vi "Add Selected Ctrl Properties.vi"(11 "Data Cluster In":T1) -> (0 "New data?":bool, 3 "Data Cluster out":T1)   [LabVIEW 2021, in "Control Property Tree.lvlib"]
uses:
  Control Property Tree.lvlib
  Module Data--cluster.ctl
  Ctrl Properties Map Data.ctl
  Property array.ctl
  Selected Ctrls - List of Controls.ctl
  Selected Ctrls - List of Properties.ctl
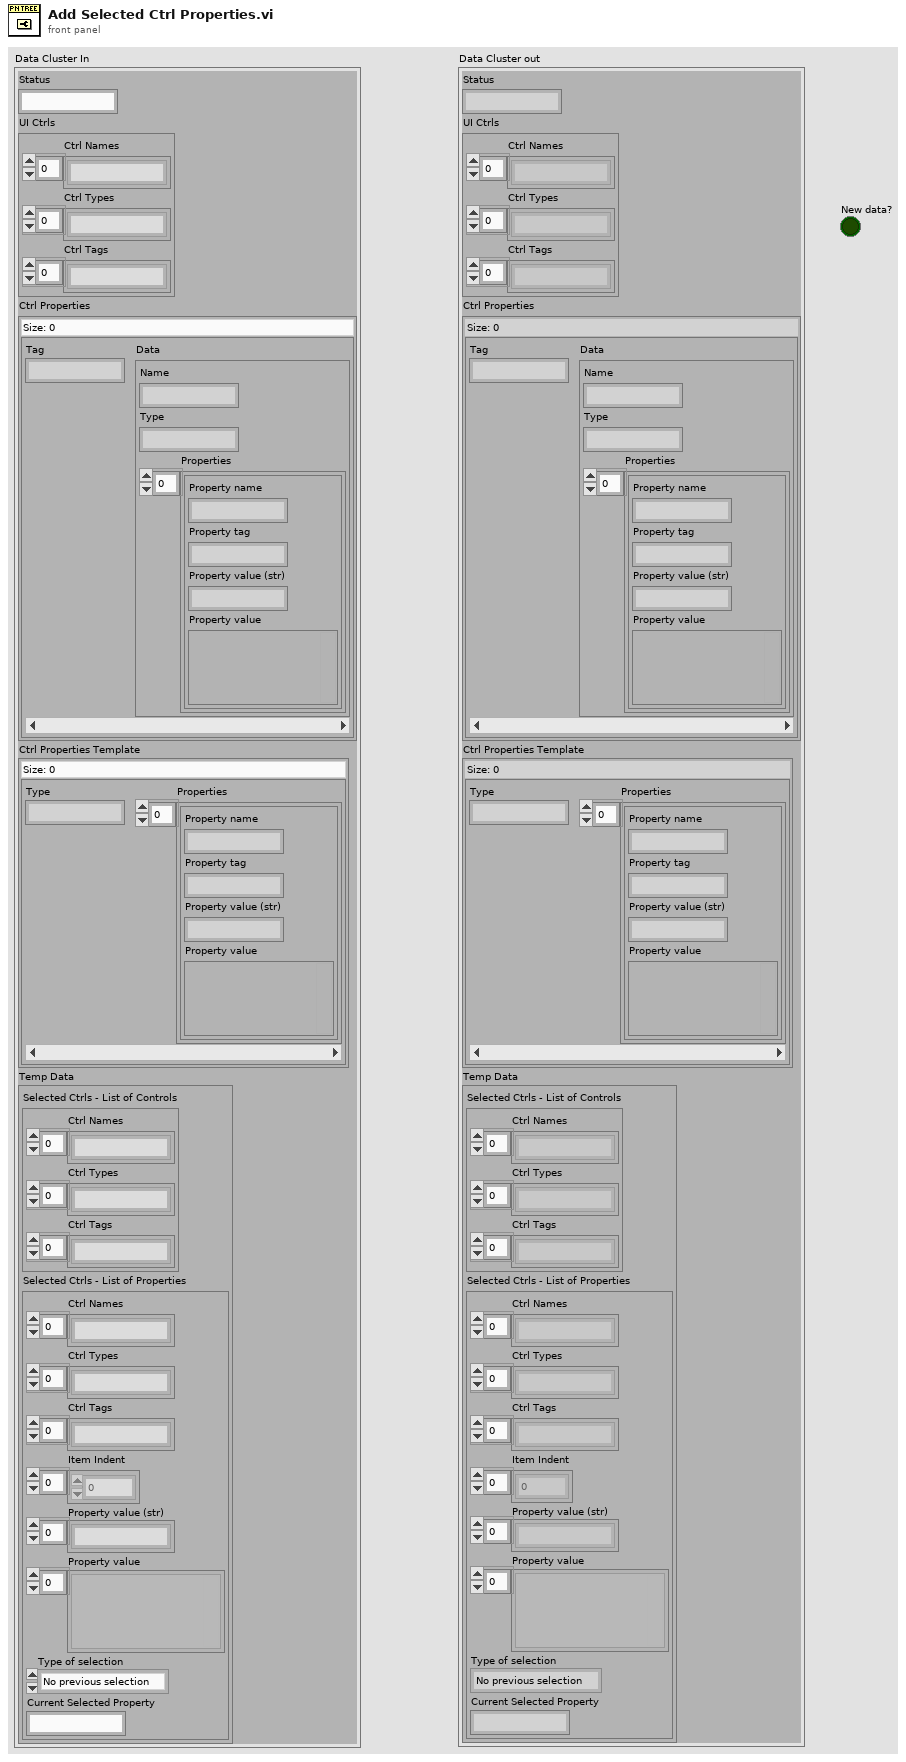
[diagram p1: front panel]
types:
  T1 = typedef "Control Property Tree.lvlib/Module Data--cluster.ctl" = cluster{"Status":string, "UI Ctrls":cluster{"Ctrl Names":string[], "Ctrl Types":string[], "Ctrl Tags":string[]}, "Ctrl Properties":map{string, T2}, "Ctrl Properties Template":map{string, T3}, "Temp Data":cluster{"Selected Ctrls - List of Controls":T4, "Selected Ctrls - List of Properties":T5}}
  T2 = typedef "Control Property Tree.lvlib/Ctrl Properties Map Data.ctl" = cluster{"Name":string, "Type":string, "Properties":T3}
  T3 = typedef "Control Property Tree.lvlib/Property array.ctl" = cluster{"Property name":string, "Property tag":string, "Property value (str)":string, "Property value":variant}[]
  T4 = typedef "Control Property Tree.lvlib/Selected Ctrls - List of Controls.ctl" = cluster{"Ctrl Names":string[], "Ctrl Types":string[], "Ctrl Tags":string[]}
  T5 = typedef "Control Property Tree.lvlib/Selected Ctrls - List of Properties.ctl" = cluster{"Ctrl Names":string[], "Ctrl Types":string[], "Ctrl Tags":string[], "Item Indent":i32[], "Property value (str)":string[], "Property value":variant[], "Type of selection":enum16{"No previous selection", "Control selected", "Property selected"}, "Current Selected Property":string}
  T6 = cluster{"Property name":string, "Property tag":string, "Property value (str)":string, "Property value":variant}
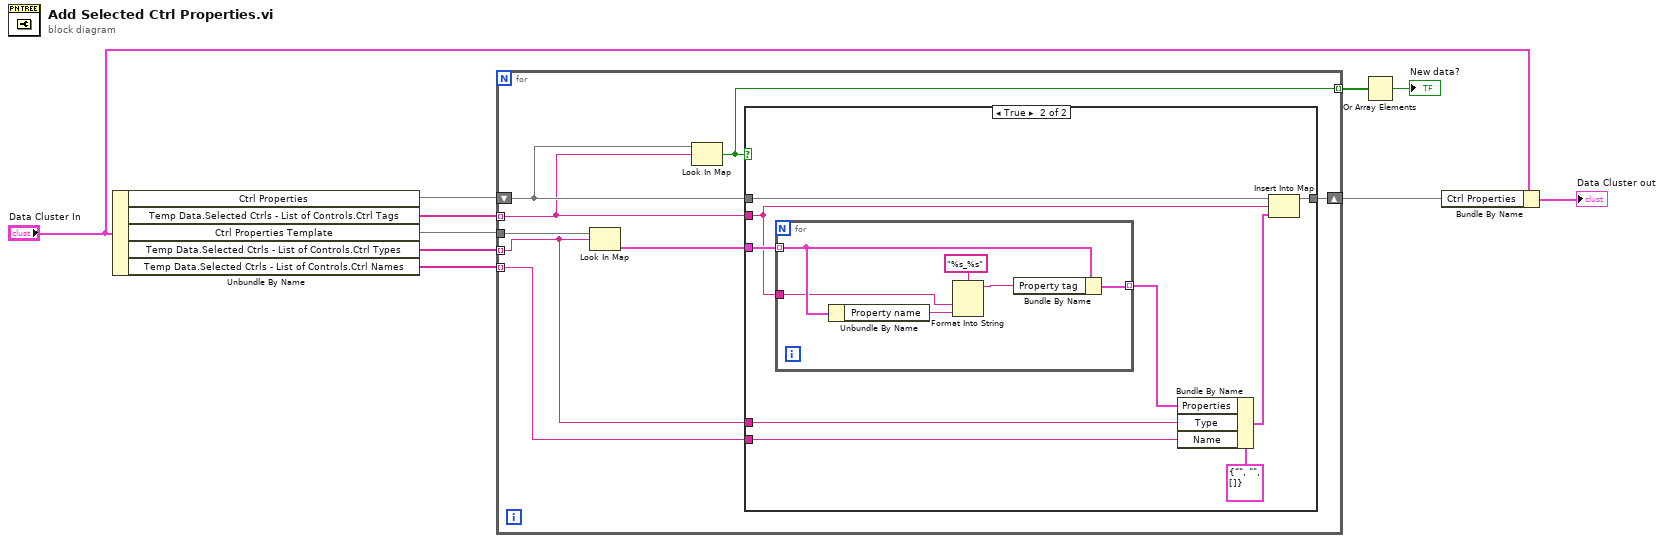
[diagram p0: block diagram]
diagram:
  n1 = Unbundle By Name("Data Cluster In") -> ("Ctrl Properties"=w7:map{string, T2}, "Temp Data.Selected Ctrls - List of Controls.Ctrl Tags"=w6:string[], "Ctrl Properties Template"=w8:map{string, T3}, "Temp Data.Selected Ctrls - List of Controls.Ctrl Types"=w10:string[], "Temp Data.Selected Ctrls - List of Controls.Ctrl Names"=w9:string[])
  n2 = for {
    tunnel: w10 -> [w16] mode=indexing
    tunnel: w9 -> [w15] mode=indexing
    tunnel: w8 -> [w18]
    tunnel: w6 -> [w12] mode=indexing
    shift-right: [w14] -> w4
    shift-left: w7 -> [w13]
    tunnel: [w11] -> w2 mode=indexing
    n3 = Look In Map(map=w18, key=w16) -> (value=w17:T3)  [unwired: 1 in, 1 out]
    n4 = Look In Map(map=w13, key=w12) -> (key not found?=w11:bool)  [unwired: 1 in, 1 out]
    n5 = case shown="True" w11 {
      tunnel: w13 -> [w19 w28]
      tunnel: w12 -> [_ w21]
      tunnel: w17 -> [_ w22]
      tunnel: w16 -> [_ w27]
      tunnel: w15 -> [_ w26]
      tunnel: [w19 w24] -> w14
      frame False {
      }
      frame True {
        n6 = for {
          tunnel: w22 -> [w34] mode=indexing
          tunnel: w21 -> [w31]
          tunnel: [w29] -> w20 mode=indexing
          n7 = Unbundle By Name(w34) -> ("Property name"=w32:string)
          n8 = Format Into String(format string="%s_%s", w31, w32) -> (resulting string=w30:string)  [unwired: 2 in, 1 out]
          n9 = Bundle By Name(cluster=w34, "Property tag"=w30) -> (w29:T6)
        }
        n10 = Bundle By Name(cluster=T2 {"Name"="", "Type"="", "Properties"=[]} ("Data"), "Properties"=w20, "Type"=w27, "Name"=w26) -> (w25:T2)
        n11 = Insert Into Map(map in=w28, key=w21, value=w25) -> (map out=w24:map{string, T2})  [unwired: 2 out]
      }
    }
  }
  n12 = Or Array Elements(Boolean array=w2) -> (logical OR=→"New data?":bool)
  n13 = Bundle By Name(cluster="Data Cluster In", "Ctrl Properties"=w4) -> (→"Data Cluster out":T1)
